vi "Receive Communication from Target.vi"(8 "error in (no error)":errorcluster, 11 "Program Data":T1={"Measurements"={"Channel 0"="Channel 0", "RMS 0"="RMS:", "Vp-p 0"="Vp-p:", "Freq 0"="Freq:", "Channel 1"="Channel 1", "RMS 1"="RMS:", "Vp-p 1"="Vp-p:", "Freq 1"="Freq:", "Cursors"="Channel 0", "C1"="Channel 0", "C2"="Channel 0", "dT"="Channel 0"}, "C1"={"Name"="", "X"=0.0, "Y"=0.0}, "C2"={"Name"="", "X"=0.0, "Y"=0.0}, "Com"={"Connection Info"={"connection ID"=refnum, "meta data"=[]}, "Connected?"=FALSE, "IP"=""}, "Continuous?"=FALSE, "Scope Data"={"AI0"=[], "AI1"=[]}, "Wave Parameters"={"Frequency (Hz)"=5.0, "Phase offset (deg)"=0.0, "Vpeak (V)"=5.0, "Offset (V)"=0.0, "Waveform"=enum."Sine", "Channel"=enum."CH0"}, "Acquire?"=FALSE, "Measure Ref"=refnum, "CH0"={"Channel"=enum."AI 0", "Enable"=FALSE, "Volts/Div"=0, "Vertical Position (Div)"=0.0}, "CH1"={"Channel"=enum."AI 0", "Enable"=FALSE, "Volts/Div"=0, "Vertical Position (Div)"=0.0}, "CH0 Params"={"V/Div"=0.0, "Units"=""}, "CH1 Params"={"V/Div"=0.0, "Units"=""}, "Time"={"Time/Div"=0.0}, "dT"=0.0, "FGen"={"Offset (V)"=0.0, "Enable Sweep"=FALSE, "Start Frequency (Hz)"=0.0, "Stop Frequency (Hz)"=0.0, "Step (Hz)"=0.0, "Step Interval (ms)"=0.0, "Current Freq (Hz)"=0.0, "Run"=FALSE}} {"Time"."Time/Div" min=0.0 max=16.0 step=1.0 scale=0.0..12.0; "CH1"."Vertical Position (Div)" min=-5.0 max=5.0 step=0.1 scale=-5.0..5.0; "CH1"."Volts/Div" min=0 max=8 step=1 scale=0.0..8.0; "CH0"."Vertical Position (Div)" min=-5.0 max=5.0 step=0.1 scale=-5.0..5.0; "CH0"."Volts/Div" min=0 max=8 step=1 scale=0.0..8.0; "Wave Parameters"."Phase offset (deg)" format="%#_6p"; "Wave Parameters"."Frequency (Hz)" format="%#_6p"}) -> (0 "error out":errorcluster, 3 "Program Data Out":T1={"Measurements"={"Channel 0"="Channel 0", "RMS 0"="RMS:", "Vp-p 0"="Vp-p:", "Freq 0"="Freq:", "Channel 1"="Channel 1", "RMS 1"="RMS:", "Vp-p 1"="Vp-p:", "Freq 1"="Freq:", "Cursors"="Channel 0", "C1"="Channel 0", "C2"="Channel 0", "dT"="Channel 0"}, "C1"={"Name"="", "X"=0.0, "Y"=0.0}, "C2"={"Name"="", "X"=0.0, "Y"=0.0}, "Com"={"Connection Info"={"connection ID"=refnum, "meta data"=[]}, "Connected?"=FALSE, "IP"=""}, "Continuous?"=FALSE, "Scope Data"={"AI0"=[], "AI1"=[]}, "Wave Parameters"={"Frequency (Hz)"=5.0, "Phase offset (deg)"=0.0, "Vpeak (V)"=5.0, "Offset (V)"=0.0, "Waveform"=enum."Sine", "Channel"=enum."CH0"}, "Acquire?"=FALSE, "Measure Ref"=refnum, "CH0"={"Channel"=enum."AI 0", "Enable"=FALSE, "Volts/Div"=0, "Vertical Position (Div)"=0.0}, "CH1"={"Channel"=enum."AI 0", "Enable"=FALSE, "Volts/Div"=0, "Vertical Position (Div)"=0.0}, "CH0 Params"={"V/Div"=0.0, "Units"=""}, "CH1 Params"={"V/Div"=0.0, "Units"=""}, "Time"={"Time/Div"=0.0}, "dT"=0.0, "FGen"={"Offset (V)"=0.0, "Enable Sweep"=FALSE, "Start Frequency (Hz)"=0.0, "Stop Frequency (Hz)"=0.0, "Step (Hz)"=0.0, "Step Interval (ms)"=0.0, "Current Freq (Hz)"=0.0, "Run"=FALSE}} {"Time"."Time/Div" min=0.0 max=16.0 step=1.0 scale=0.0..12.0; "CH1"."Vertical Position (Div)" min=-5.0 max=5.0 step=0.1 scale=-5.0..5.0; "CH1"."Volts/Div" min=0 max=8 step=1 scale=0.0..8.0; "CH0"."Vertical Position (Div)" min=-5.0 max=5.0 step=0.1 scale=-5.0..5.0; "CH0"."Volts/Div" min=0 max=8 step=1 scale=0.0..8.0; "Wave Parameters"."Phase offset (deg)" format="%#_6p"; "Wave Parameters"."Frequency (Hz)" format="%#_6p"})   [LabVIEW 2018]
uses:
  Controls/Program Data.ctl
  Controls/Measurements.ctl
  Controls/Channel Measurement String Control.ctl
  Controls/Cursor Info.ctl
  Controls/Communication Cluster.ctl
  <vilib>/NI/STM/TCP/TCP Connection Info.ctl
  <vilib>/NI/STM/SubVIs/MetaDataElement.ctl
  Scope Data.ctl
  Program Files (x86)/National Instruments/LabVIEW 2018/ProjectTemplates/Source/myRIO/Oscilloscope/myRIO v1.1/Real-Time/Controls/Wave Parameters.ctl
  Program Files (x86)/National Instruments/LabVIEW 2018/ProjectTemplates/Source/myRIO/Oscilloscope/myRIO v1.1/Real-Time/Controls/Waveform Enum.ctl
  Program Files (x86)/National Instruments/LabVIEW 2018/ProjectTemplates/Source/myRIO/Oscilloscope/myRIO v1.1/Real-Time/Controls/Channel Selector.ctl
  Controls/Channel Settings.ctl
  Controls/Analog Input Selector.ctl
  Controls/Knob.ctl
  Controls/Vertical Position.ctl
  Controls/Channel Parameters.ctl
  Controls/Time Selector.ctl
  Controls/Time Knob.ctl
  Controls/FGen Desktop Configuration.ctl
  <vilib>/NI/STM/TCP/TCP Read Options.ctl
  <vilib>/NI/STM/TCP/Read Message (TCP).vi
  <vilib>/NI/STM/NI STM.lvlib
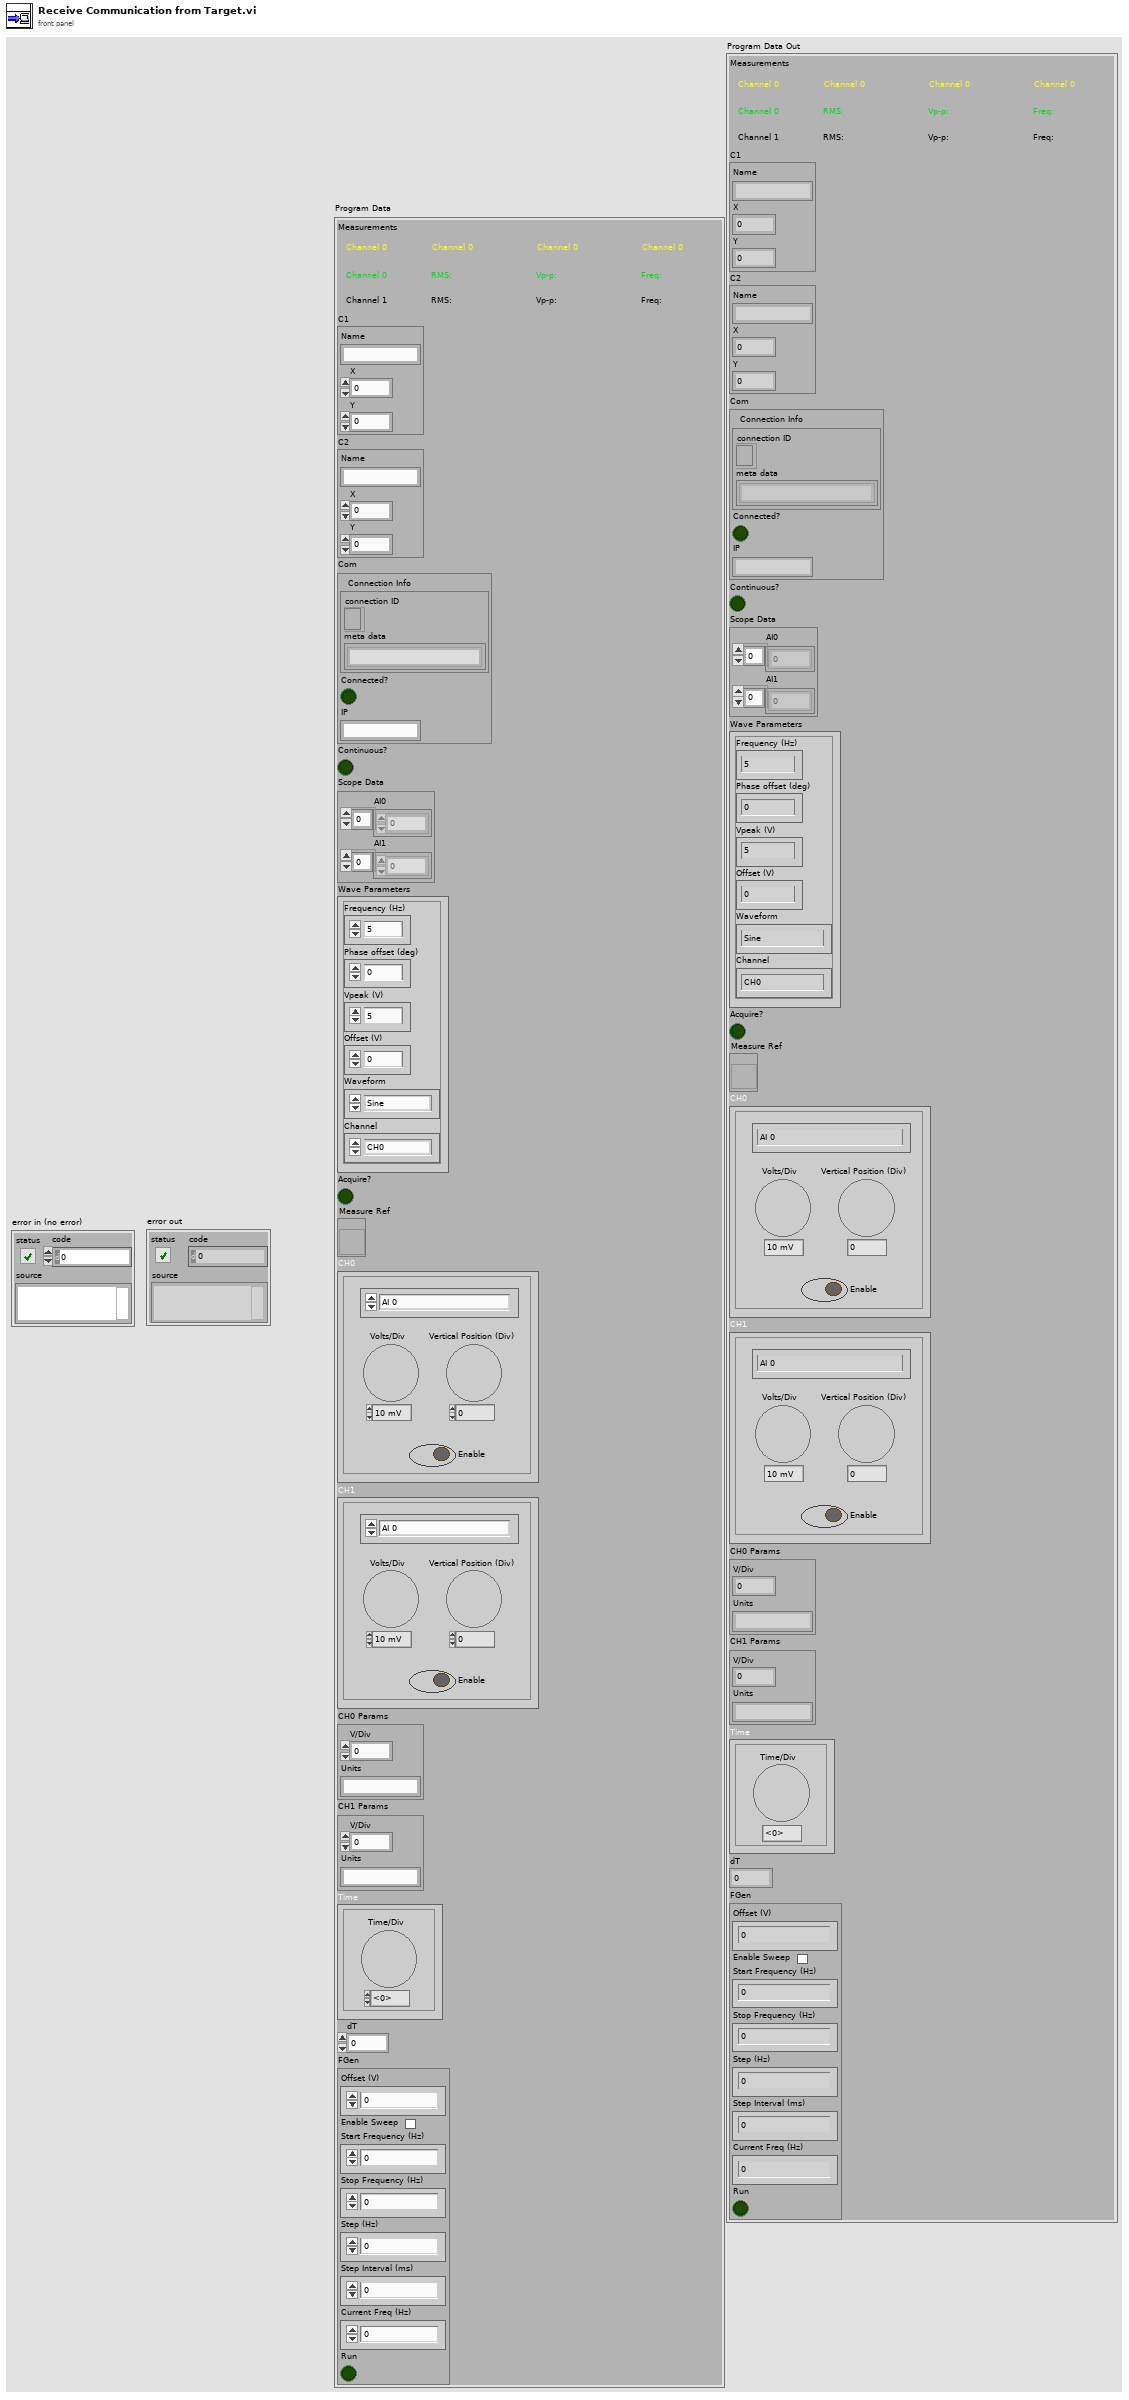
[diagram p1: front panel]
types:
  T1 = typedef "Program Data.ctl" = cluster{"Measurements":T2, "C1":T4, "C2":T4, "Com":T5, "Continuous?":bool, "Scope Data":T8, "Wave Parameters":T9, "Acquire?":bool, "Measure Ref":refnum<vi>, "CH0":T12, "CH1":T12, "CH0 Params":T16, "CH1 Params":T16, "Time":T17, "dT":dbl, "FGen":T19}
  T2 = typedef "Measurements.ctl" = cluster{"Channel 0":T3, "RMS 0":T3, "Vp-p 0":T3, "Freq 0":T3, "Channel 1":T3, "RMS 1":T3, "Vp-p 1":T3, "Freq 1":T3, "Cursors":T3, "C1":T3, "C2":T3, "dT":T3}
  T3 = typedef "Channel Measurement String Control.ctl" = string
  T4 = typedef "Cursor Info.ctl" = cluster{"Name":string, "X":dbl, "Y":dbl}
  T5 = typedef "Communication Cluster.ctl" = cluster{"Connection Info":T6, "Connected?":bool, "IP":string}
  T6 = typedef "NI STM.lvlib/TCP Connection Info.ctl" = cluster{"connection ID":refnum<k5>, "meta data":T7[]}
  T7 = typedef "NI STM.lvlib/MetaDataElement.ctl" = string
  T8 = typedef "Scope Data.ctl" = cluster{"AI0":dbl[], "AI1":dbl[]}
  T9 = typedef "Wave Parameters.ctl" = cluster{"Frequency (Hz)":dbl, "Phase offset (deg)":dbl, "Vpeak (V)":dbl, "Offset (V)":dbl, "Waveform":T10, "Channel":T11}
  T10 = typedef "Waveform Enum.ctl" = enum16{"Sine", "Square"}
  T11 = typedef "Channel Selector.ctl" = enum16{"CH0", "CH1"}
  T12 = typedef "Channel Settings.ctl" = cluster{"Channel":T13, "Enable":bool, "Volts/Div":T14, "Vertical Position (Div)":T15}
  T13 = typedef "Analog Input Selector.ctl" = enum16{"AI 0", "AI 1"}
  T14 = typedef "Knob.ctl" = i32
  T15 = typedef "Vertical Position.ctl" = dbl
  T16 = typedef "Channel Parameters.ctl" = cluster{"V/Div":dbl, "Units":string}
  T17 = typedef "Time Selector.ctl" = cluster{"Time/Div":T18}
  T18 = typedef "Time Knob.ctl" = dbl
  T19 = typedef "FGen Desktop Configuration.ctl" = cluster{"Offset (V)":dbl, "Enable Sweep":bool, "Start Frequency (Hz)":dbl, "Stop Frequency (Hz)":dbl, "Step (Hz)":dbl, "Step Interval (ms)":dbl, "Current Freq (Hz)":dbl, "Run":bool}
  T20 = typedef "NI STM.lvlib/TCP Read Options.ctl" = cluster{"ignore timeout error":bool, "timeout ms (1000)":i32}
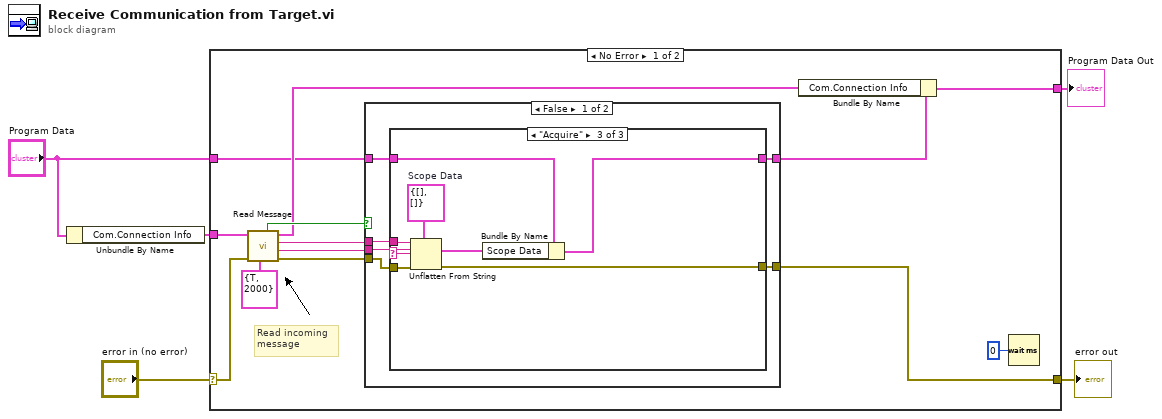
[diagram p0: block diagram]
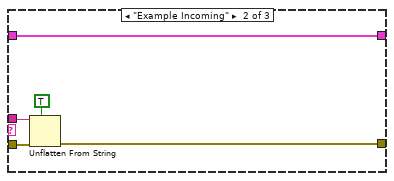
[diagram p3: hidden frame]
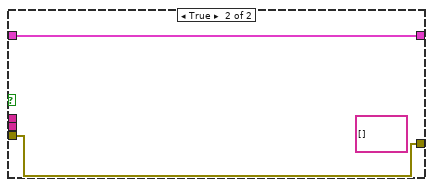
[diagram p4: hidden frame]
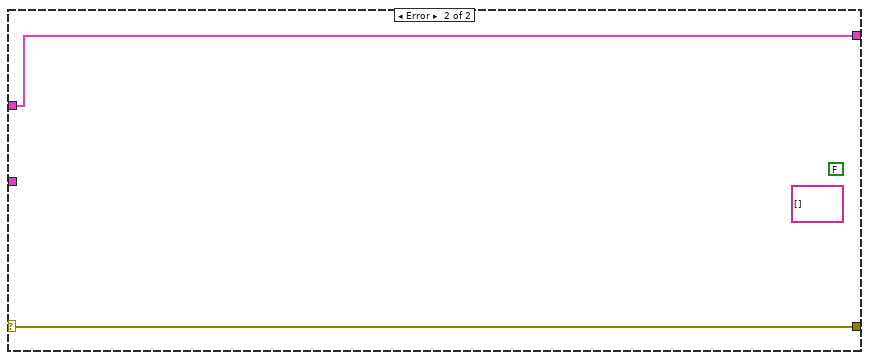
[diagram p5: hidden frame]
diagram:
  n1 = Unbundle By Name("Program Data") -> ("Com.Connection Info"=w3:T6)
  n2 = case shown="No Error" "error in (no error)" {
    selector: "error in (no error)" -> [w13 w42]
    tunnel: w3 -> [w7 _]
    tunnel: [w14 w42] -> w5
    tunnel: "Program Data" -> [w10 w41]
    tunnel: [w9 w41] -> w1
    frame No Error {
      # "Read incoming\nmessage"
      n3 = call-poly <vilib>:"Read Message.vi"("options"=T20 {"ignore timeout error"=TRUE, "timeout ms (1000)"=2000} ("Options"), "error in"=w13, "connection info in"=w7) -> ("error out"=w15:errorcluster, "name"=w18:T7, "data string"=w17:string, "connection info out"=w11:T6, "timed out?"=w16:bool)  [unwired: 4 out]
      n4 = case shown="False" w16 {
        tunnel: w18 -> [w23 _]
        tunnel: w17 -> [w24 _]
        tunnel: w15 -> [w22 w40]
        tunnel: [w21 w40] -> w14
        tunnel: w10 -> [w20 w39]
        tunnel: [w19 w39] -> w8
        frame False {
          n5 = case shown="\"Acquire\"" w23 {
            tunnel: w24 -> [_ w30 w37]
            tunnel: w22 -> [w26 w31 w38]
            tunnel: [w26 w27 w36] -> w21
            tunnel: w20 -> [w25 w28 w34]
            tunnel: [w25 w28 w33] -> w19
            frame Default {
            }
            frame "Example Incoming" {
              n6 = Unflatten From String(type=TRUE, binary string=w30, error in (no error)=w31) -> (error out=w27:errorcluster)  [unwired: 2 in, 2 out]
            }
            frame "Acquire" {
              w35 = T8 {"AI0"=[], "AI1"=[]}  # Scope Data
              n7 = Unflatten From String(type=w35, binary string=w37, error in (no error)=w38) -> (value=w32:T8, error out=w36:errorcluster)  [unwired: 2 in, 1 out]
              n8 = Bundle By Name(cluster=w34, "Scope Data"=w32) -> (w33:T1)
            }
          }
        }
        frame True {
          (unwired) string[][] [] ("Test Result")
        }
      }
      n9 = Bundle By Name(cluster=w8, "Com.Connection Info"=w11) -> (w9:T1)
      n10 = Wait (ms)(milliseconds to wait=u32 0) -> ()  [unwired: 1 out]
    }
    frame Error {
      (unwired) FALSE
      (unwired) string[][] [] ("Test Result")
    }
  }
  "error out" <- w5
  "Program Data Out" <- w1
